vi "RDS Create Subscription.vi"(8 "error in (no error)":errorcluster, 10 "Subscribed IDs":T1[](array[typedef]), 11 "RDS Child Enqueuer":refnum<class "Message Enqueuer.lvclass">) -> (0 "error out":errorcluster, 3 "RDS Router Subscription out":refnum<class "RDS Router Subscription.lvclass">)   [LabVIEW 2015, in "RDS Abstracts.lvlib" / "RDS Router Actor.lvlib" / "RDS Router Subscription.lvclass"]
uses:
  RDS Router Subscription.lvclass
  <vilib>/ActorFramework/Message Enqueuer/Message Enqueuer.lvclass
  Libraries/RDS Framework/RDS Message ID.ctl
  RDS Router Subscription.lvclass/RDS Router Subscription.ctl
  Libraries/RDS Child Messages/RDS Child Messages.lvlib
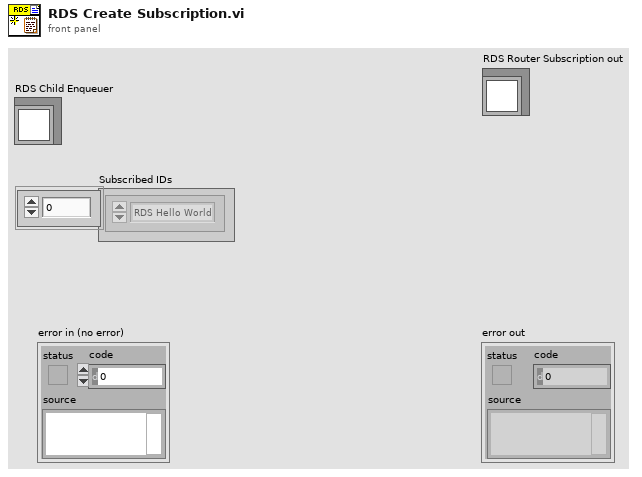
[diagram p1: front panel]
types:
  T1 = typedef "RDS Child Messages.lvlib/RDS Message ID.ctl" = enum16{"RDS Hello World", "String Message", "AIP_Status", "AIP_Command", "GPS_Data", "MCB_Command", "MCB_Status", "Compass_Data", "Depth_Data", "Battery_Data", "Contoller_State", "Set_Mag_Dev", "BTB_Shutdown", "State_Sample_Request", "State_Sample", "PID_Gains_Set", "Helm_Limiter_Set", "Helm_Heading_Command", "Helm_Steering_Command", "Helm_Status", "Controller_Message", "AIP_Set_Min_Depth", "Mission_Controller_State", "Mission_Upload", "Mission_Set_Op_and_Run", "Mission_Settings_Set"}
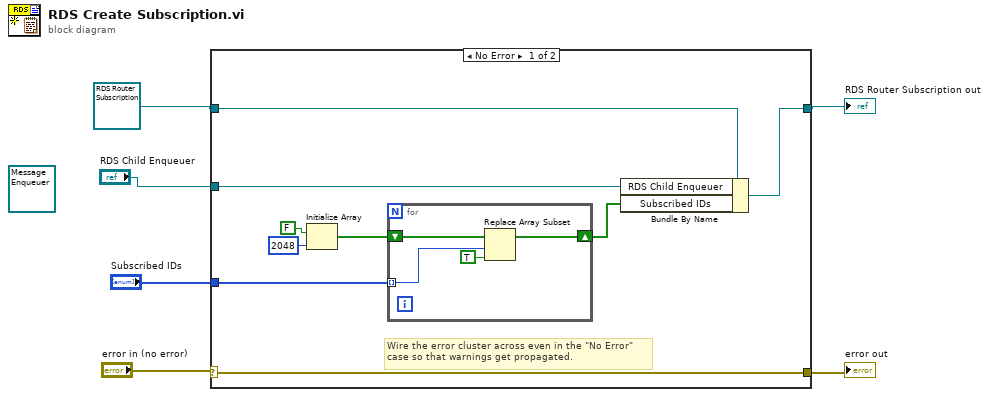
[diagram p0: block diagram]
diagram:
  (unwired) refnum<class "Message Enqueuer.lvclass"> refnum ("RDS Child Enqueuer")
  n1 = case shown="No Error" "error in (no error)" {
    selector: "error in (no error)" -> [w15 w21]
    tunnel: [w15 w21] -> w2
    tunnel: [w9 w20] -> w6
    tunnel: refnum<class "RDS Router Subscription.lvclass"> refnum ("RDS Router Subscription in") -> [w10 w20]
    tunnel: "Subscribed IDs" -> [w12 _]
    tunnel: "RDS Child Enqueuer" -> [w7 _]
    frame No Error {
      # "Wire the error cluster across even in the \"No Error\"\ncase so that warnings get propagated."
      n2 = Initialize Array(FALSE, 2048 ("dimension size")) -> (w11:bool[])
      n3 = for {
        tunnel: w12 -> [w18] mode=indexing
        shift-right: [w16] -> w8
        shift-left: w11 -> [w19]
        n4 = Replace Array Subset(array=w19, new element=TRUE ("new element/subarray"), index=w18) -> (w16:bool[])
      }
      n5 = Bundle By Name(cluster=w10, "RDS Child Enqueuer"=w7, "Subscribed IDs"=w8) -> (w9:refnum<class "RDS Router Subscription.lvclass">)
    }
    frame Error {
    }
  }
  "error out" <- w2
  "RDS Router Subscription out" <- w6
